vi "Data_Save_Initialisation.vi"() -> (2 "Initialisation":string[](array[string]))   [LabVIEW 2017]
uses:
  Ctrls/CSV_Data.ctl
panel:
  in  "Data in":T1
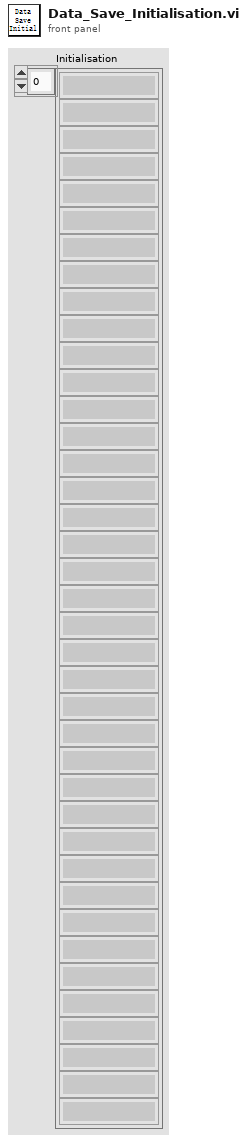
[diagram p1: front panel]
types:
  T1 = typedef "CSV_Data.ctl" = cluster{"Initialisation":cluster{"LMT - Connect UUT (con COM)":cluster{"Vaule":string, "Status":string, "Step Time":dbl}, "LMT - Software Version (rrel)":cluster{"Vaule":string, "Status":string, "Step Time":dbl}, "LMT - Write SKU file (wskuc)":cluster{"Vaule":string, "Status":string, "Step Time":dbl}, "LMT - SKU file name":cluster{"Vaule":string, "Status":string, "Step Time":dbl}, "LMT Connect UUT - Error Log":cluster{"Vaule":string, "Status":string, "Step Time":dbl}, "5.3.2.1 Connect UUT DDM":cluster{"Vaule":string, "Status":string, "Step Time":dbl}, "Connect UUT DDM - Error Log":cluster{"Vaule":string, "Status":string, "Step Time":dbl}, "5.3.2.8 Read DDM EOL Timestamp":cluster{"Vaule":string, "Status":string, "Step Time":dbl}, "5.3.2.8 Read DDM EOL Timestamp - Mode":cluster{"Vaule":string, "Status":string, "Step Time":dbl}, "5.3.2.8 Read DDM EOL Timestamp - Timestamp":cluster{"Vaule":string, "Status":string, "Step Time":dbl}, "5.3.2.8 Read DDM EOL Timestamp - Rig ID":cluster{"Vaule":string, "Status":string, "Step Time":dbl}, "5.3.2.8 Read DDM EOL Timestamp - Passmark ID":cluster{"Vaule":string, "Status":string, "Step Time":dbl}, "5.3.2.8 Read DDM EOL Timestamp - Passmark Rev":cluster{"Vaule":string, "Status":string, "Step Time":dbl}, "Read DDM EOL Timestamp - Error Log":cluster{"Vaule":string, "Status":string, "Step Time":dbl}, "5.3.2.2 Read DDM SW Version before flashing":cluster{"Vaule":string, "Status":string, "Step Time":dbl}, "5.3.2.2 Software Version before flashing":cluster{"Vaule":string, "Status":string, "Step Time":dbl}, "Read DDM SW Version before flashing - Error Log":cluster{"Vaule":string, "Status":string, "Step Time":dbl}, "5.3.2.7 Read Hardware Serial":cluster{"Vaule":string, "Status":string, "Step Time":dbl}, "Read Hardware Serial - Error Log":cluster{"Vaule":string, "Status":string, "Step Time":dbl}, "Read DDM SN from UUT":cluster{"Vaule":string, "Status":string, "Step Time":dbl}, "UUT DDM SN":cluster{"Vaule":string, "Status":string, "Step Time":dbl}, "Compare Length":cluster{"Vaule":string, "Status":string, "Step Time":dbl}, "Compare DDM SN with MES SN":cluster{"Vaule":string, "Status":string, "Step Time":dbl}, "Check DDM SN - Error Log":cluster{"Vaule":string, "Status":string, "Step Time":dbl}, "5.3.6.2.2 Backup File Data - CAL":cluster{"Vaule":string, "Status":string, "Step Time":dbl}, "5.3.6.2.2 Backup Data Response - CAL":cluster{"Vaule":string, "Status":string, "Step Time":dbl}, "5.3.2.3 Flash Firmware Version":cluster{"Vaule":string, "Status":string, "Step Time":dbl}, "5.3.2.4 Wait Timeout":cluster{"Vaule":string, "Status":string, "Step Time":dbl}, "5.3.2.5 Check SW Version":cluster{"Vaule":string, "Status":string, "Step Time":dbl}, "5.3.2.5 Flashing firmware file name":cluster{"Vaule":string, "Status":string, "Step Time":dbl}, "Flash Firmware Version - Error Log":cluster{"Vaule":string, "Status":string, "Step Time":dbl}, "5.3.2a.1 Disconnect UUT":cluster{"Vaule":string, "Status":string, "Step Time":dbl}, "Disconnect UUT - Error Log":cluster{"Vaule":string, "Status":string, "Step Time":dbl}, "5.3.2a.3 Connect UUT UI":cluster{"Vaule":string, "Status":string, "Step Time":dbl}, "Connect UUT UI - Error Log":cluster{"Vaule":string, "Status":string, "Step Time":dbl}, "5.3.2a.4 Flash Firmware Version":cluster{"Vaule":string, "Status":string, "Step Time":dbl}, "5.3.2a.4 Wait Timeout":cluster{"Vaule":string, "Status":string, "Step Time":dbl}, "5.3.2a.4 Check SW Version":cluster{"Vaule":string, "Status":string, "Step Time":dbl}, "5.3.2a.5 Flashing firmware file name":cluster{"Vaule":string, "Status":string, "Step Time":dbl}, "Flash Firmware Version - Error Log":cluster{"Vaule":string, "Status":string, "Step Time":dbl}, "5.3.2.6 Read DDM SW Version after flashing":cluster{"Vaule":string, "Status":string, "Step Time":dbl}, "5.3.2.6 Check DDM SW Version after flashing":cluster{"Vaule":string, "Status":string, "Step Time":dbl}, "Read DDM SW Version after flashing - Error Log":cluster{"Vaule":string, "Status":string, "Step Time":dbl}, "5.3.2.10 Set SKU Config Status":cluster{"Vaule":string, "Status":string, "Step Time":dbl}, "5.3.2.10 Set SKU Config":cluster{"Vaule":string, "Status":string, "Step Time":dbl}, "5.3.2.10 Set SKU Config File Name":cluster{"Vaule":string, "Status":string, "Step Time":dbl}, "Set SKU Config - Error Log":cluster{"Vaule":string, "Status":string, "Step Time":dbl}, "5.3.2.10 Ready Status":cluster{"Vaule":string, "Status":string, "Step Time":dbl}, "Ready Status - Error Log":cluster{"Vaule":string, "Status":string, "Step Time":dbl}, "5.3.2.12 Set Device Mode to EOL":cluster{"Vaule":string, "Status":string, "Step Time":dbl}, "5.3.2.12 DDM EOL mode":cluster{"Vaule":string, "Status":string, "Step Time":dbl}, "Set Device Mode - Error Log":cluster{"Vaule":string, "Status":string, "Step Time":dbl}, "5.3.4.34 Wait 1s":cluster{"Vaule":string, "Status":string, "Step Time":dbl}, "5.3.2.13 DDM Parameter - Voltage":cluster{"Vaule":string, "Status":string, "Step Time":dbl}, "5.3.2.13 DDM Parameter - Current":cluster{"Vaule":string, "Status":string, "Step Time":dbl}, "5.3.2.13 DDM Parameter - Power":cluster{"Vaule":string, "Status":string, "Step Time":dbl}, "5.3.2.13 DDM Parameter - Speed":cluster{"Vaule":string, "Status":string, "Step Time":dbl}, "5.3.2.13 DDM Parameter - Pressure":cluster{"Vaule":string, "Status":string, "Step Time":dbl}, "5.3.2.14 Tester Parameter - Voltage":cluster{"Vaule":string, "Status":string, "Step Time":dbl}, "5.3.2.14 Tester Parameter - Current":cluster{"Vaule":string, "Status":string, "Step Time":dbl}, "5.3.2.14 Tester Parameter - Power":cluster{"Vaule":string, "Status":string, "Step Time":dbl}, "5.3.2.14 Tester Parameter - Ambient Pressure":cluster{"Vaule":string, "Status":string, "Step Time":dbl}, "5.3.2.14 Tester Parameter - Ambient Temperature":cluster{"Vaule":string, "Status":string, "Step Time":dbl}, "5.3.2.14 Tester Parameter - Pressure Box":cluster{"Vaule":string, "Status":string, "Step Time":dbl}, "5.3.2.14 Tester Parameter - Reference Ambient Pressure":cluster{"Vaule":string, "Status":string, "Step Time":dbl}, "5.3.2.15 Calculated Parameter - DDM Pressure Corrected":cluster{"Vaule":string, "Status":string, "Step Time":dbl}, "5.3.2.15 Calculated Parameter - DDM Real Power":cluster{"Vaule":string, "Status":string, "Step Time":dbl}, "5.3.2.15 Calculated Parameter - Delta V":cluster{"Vaule":string, "Status":string, "Step Time":dbl}, "Get and Check Parameter - Error Log":cluster{"Vaule":string, "Status":string, "Step Time":dbl}}, "BEMF_Calibration":cluster{"5.3.3.0 Read BEMF ambient temperature":cluster{"Vaule":string, "Status":string, "Step Time":dbl}, "5.3.3.0 Calibration Result - eol_cold_bemf_temp":cluster{"Vaule":string, "Status":string, "Step Time":dbl}, "Read BEMF ambient temperature - Error Log":cluster{"Vaule":string, "Status":string, "Step Time":dbl}, "5.3.3.0 Set ambient temp to DDM":cluster{"Vaule":string, "Status":string, "Step Time":dbl}, "5.3.3.0 DDM Ambient Temp":cluster{"Vaule":string, "Status":string, "Step Time":dbl}, "Set ambient temp to DDM - Error Log":cluster{"Vaule":string, "Status":string, "Step Time":dbl}, "5.3.4.2 Restriction Plate Diameter":cluster{"Vaule":string, "Status":string, "Step Time":dbl}, "5.3.4.2 BEMF CAL - Put 13mm Restriction Plate":cluster{"Vaule":string, "Status":string, "Step Time":dbl}, "Put Restriction Plate - Error Log":cluster{"Vaule":string, "Status":string, "Step Time":dbl}, "5.3.3.1 Set - Calibrate BEMF both":cluster{"Vaule":string, "Status":string, "Step Time":dbl}, "5.3.3.1 Get - Calibrate BEMF LSI":cluster{"Vaule":string, "Status":string, "Step Time":dbl}, "5.3.3.2 Get - Calibration Result - eol_bemf_mp_cold_coef_a":cluster{"Vaule":string, "Status":string, "Step Time":dbl}, "5.3.3.2 Get - Calibration Result - eol_bemf_mp_cold_coef_b":cluster{"Vaule":string, "Status":string, "Step Time":dbl}, "5.3.3.2 Get - Calibration Result - eol_bemf_mp_cold_coef_c":cluster{"Vaule":string, "Status":string, "Step Time":dbl}, "5.3.3.2 Get - Calibration Result - eol_bemf_lsi_cold_ref_coeffs":cluster{"Vaule":string, "Status":string, "Step Time":dbl}, "5.3.3.2 Get - Calibration Result - eol_bemf_lsi_speed":cluster{"Vaule":string, "Status":string, "Step Time":dbl}, "5.3.3.2 Get - Calibration Result - eol_bemf_lsi_integral_0":cluster{"Vaule":string, "Status":string, "Step Time":dbl}, "5.3.3.2 Get - Calibration Result - eol_bemf_lsi_integral_1":cluster{"Vaule":string, "Status":string, "Step Time":dbl}, "5.3.3.2 Get - Calibration Result - eol_bemf_lsi_integral_2":cluster{"Vaule":string, "Status":string, "Step Time":dbl}, "5.3.3.2 Get - Calibration Result - eol_cold_bemf":cluster{"Vaule":string, "Status":string, "Step Time":dbl}, "5.3.3.2 Get - Calibration Result - eol_cold_bemf_fisf":cluster{"Vaule":string, "Status":string, "Step Time":dbl}, "Get - Calibrate BEMF LSI - Error Log":cluster{"Vaule":string, "Status":string, "Step Time":dbl}, "5.3.3.3 Finalise Calibration":cluster{"Vaule":string, "Status":string, "Step Time":dbl}, "5.3.3.4 Wait 1 sec":cluster{"Vaule":string, "Status":string, "Step Time":dbl}, "Finalise Calibration - Error Log":cluster{"Vaule":string, "Status":string, "Step Time":dbl}, "5.3.3.1 Get - Calibrate BEMF LSI":cluster{"Vaule":string, "Status":string, "Step Time":dbl}, "5.3.3.2 Get - Calibration Result - eol_cold_bemf":cluster{"Vaule":string, "Status":string, "Step Time":dbl}, "5.3.3.2 Get - Calibration Result - eol_cold_bemf_fisf":cluster{"Vaule":string, "Status":string, "Step Time":dbl}, "5.3.3.2 Compare -Calibration Result - eol_cold_bemf":cluster{"Vaule":string, "Status":string, "Step Time":dbl}, "5.3.3.2 Compare -Calibration Result - eol_cold_bemf_fisf":cluster{"Vaule":string, "Status":string, "Step Time":dbl}, "Get & Compare - Calibrate BEMF LSI - Error Log":cluster{"Vaule":string, "Status":string, "Step Time":dbl}}, "ECO":cluster{"5.3.3.3 Reset Power Tune":cluster{"Vaule":string, "Status":string, "Step Time":dbl}, "5.3.3.4 Reset Power Tune Value":cluster{"Vaule":string, "Status":string, "Step Time":dbl}, "Reset Power Tune - Error Log":cluster{"Vaule":string, "Status":string, "Step Time":dbl}, "5.3.3.3 Reset BEMF FISF Calibration":cluster{"Vaule":string, "Status":string, "Step Time":dbl}, "5.3.3.4 Reset BEMF FISF Calibration Value":cluster{"Vaule":string, "Status":string, "Step Time":dbl}, "Reset BEMF FISF Calibration - Error Log":cluster{"Vaule":string, "Status":string, "Step Time":dbl}, "5.3.4.2 ECO - Put 13mm Restriction Plate":cluster{"Vaule":string, "Status":string, "Step Time":dbl}, "5.3.4.2 Restriction Plate Diameter":cluster{"Vaule":string, "Status":string, "Step Time":dbl}, "Put Restriction Plate - Error Log":cluster{"Vaule":string, "Status":string, "Step Time":dbl}, "5.3.4.5 ECO - Motor ON":cluster{"Vaule":string, "Status":string, "Step Time":dbl}, "5.3.4.5 ECO - Motor ON Mode":cluster{"Vaule":string, "Status":string, "Step Time":dbl}, "ECO - Motor ON - Error Log":cluster{"Vaule":string, "Status":string, "Step Time":dbl}, "5.3.4.6 ECO - Motor Speed Stabilisation":cluster{"Vaule":string, "Status":string, "Step Time":dbl}, "5.3.4.6 ECO - Stabilisation Time":cluster{"Vaule":string, "Status":string, "Step Time":dbl}, "ECO - Motor Speed Stabilisation - Error Log":cluster{"Vaule":string, "Status":string, "Step Time":dbl}, "5.3.4.7 ECO - DDM Parameter - Voltage":cluster{"Vaule":string, "Status":string, "Step Time":dbl}, "5.3.4.7 ECO - DDM Parameter - Current":cluster{"Vaule":string, "Status":string, "Step Time":dbl}, "5.3.4.7 ECO - DDM Parameter - Power":cluster{"Vaule":string, "Status":string, "Step Time":dbl}, "5.3.4.7 ECO - DDM Parameter - Measured Power":cluster{"Vaule":string, "Status":string, "Step Time":dbl}, "5.3.4.7 ECO - DDM Parameter - Speed":cluster{"Vaule":string, "Status":string, "Step Time":dbl}, "5.3.4.7 ECO - DDM Parameter - Pressure":cluster{"Vaule":string, "Status":string, "Step Time":dbl}, "5.3.4.7 ECO - DDM Parameter - lsi magnet temp":cluster{"Vaule":string, "Status":string, "Step Time":dbl}, "5.3.4.7 ECO - DDM Parameter - fisf magnet temp":cluster{"Vaule":string, "Status":string, "Step Time":dbl}, "5.3.4.7 ECO - DDM Parameter - iir magnet temp":cluster{"Vaule":string, "Status":string, "Step Time":dbl}, "5.3.4.8 ECO - Tester Parameter - Voltage":cluster{"Vaule":string, "Status":string, "Step Time":dbl}, "5.3.4.8 ECO - Tester Parameter - Current":cluster{"Vaule":string, "Status":string, "Step Time":dbl}, "5.3.4.8 ECO - Tester Parameter - Power":cluster{"Vaule":string, "Status":string, "Step Time":dbl}, "5.3.4.8 ECO - Tester Parameter - Ambient Pressure":cluster{"Vaule":string, "Status":string, "Step Time":dbl}, "5.3.4.8 ECO - Tester Parameter - Ambient Temperature":cluster{"Vaule":string, "Status":string, "Step Time":dbl}, "5.3.4.8 ECO - Tester Parameter - Ambient Humidity":cluster{"Vaule":string, "Status":string, "Step Time":dbl}, "5.3.4.8 ECO - Tester Parameter - Pressure Box":cluster{"Vaule":string, "Status":string, "Step Time":dbl}, "5.3.4.8 ECO - Tester Parameter - Reference Ambient Pressure":cluster{"Vaule":string, "Status":string, "Step Time":dbl}, "5.3.4.9 ECO - Calculated Parameter - DDM Pressure Corrected":cluster{"Vaule":string, "Status":string, "Step Time":dbl}, "5.3.4.9 ECO - Calculated Parameter - DDM Real Power":cluster{"Vaule":string, "Status":string, "Step Time":dbl}, "5.3.4.9 ECO - Calculated Parameter - Delta V":cluster{"Vaule":string, "Status":string, "Step Time":dbl}, "5.3.4.9 ECO - Calculated Parameter - Flowrate":cluster{"Vaule":string, "Status":string, "Step Time":dbl}, "5.3.4.9 ECO - Calculated Parameter - Airwatt":cluster{"Vaule":string, "Status":string, "Step Time":dbl}, "5.3.4.9 ECO - Formula":cluster{"Vaule":string, "Status":string, "Step Time":dbl}, "ECO - Get and Check Parameter - Error Log":cluster{"Vaule":string, "Status":string, "Step Time":dbl}, "PT ECO - Power Tune Mode Status":cluster{"Vaule":string, "Status":string, "Step Time":dbl}, "PT ECO - Power Tune Set Delta Power Tune":cluster{"Vaule":string, "Status":string, "Step Time":dbl}, "PT ECO - Power Tune Index":cluster{"Vaule":string, "Status":string, "Step Time":dbl}, "PT ECO - Power Tune Delta_P":cluster{"Vaule":string, "Status":string, "Step Time":dbl}, "PT ECO - Power Tune Motor ON Status":cluster{"Vaule":string, "Status":string, "Step Time":dbl}, "PT ECO - Power Tune Motor ON Mode":cluster{"Vaule":string, "Status":string, "Step Time":dbl}, "PT ECO - Power Tune Stabilisation Time Status":cluster{"Vaule":string, "Status":string, "Step Time":dbl}, "PT ECO - Power Tune Stabilisation Delay Time":cluster{"Vaule":string, "Status":string, "Step Time":dbl}, "PT ECO - DDM Parameter - Voltage":cluster{"Vaule":string, "Status":string, "Step Time":dbl}, "PT ECO - DDM Parameter - Current":cluster{"Vaule":string, "Status":string, "Step Time":dbl}, "PT ECO - DDM Parameter - Power":cluster{"Vaule":string, "Status":string, "Step Time":dbl}, "PT ECO - DDM Parameter - Measured Power":cluster{"Vaule":string, "Status":string, "Step Time":dbl}, "PT ECO - DDM Parameter - Speed":cluster{"Vaule":string, "Status":string, "Step Time":dbl}, "PT ECO - DDM Parameter - Pressure":cluster{"Vaule":string, "Status":string, "Step Time":dbl}, "PT ECO - DDM Parameter - lsi magnet temp":cluster{"Vaule":string, "Status":string, "Step Time":dbl}, "PT ECO - DDM Parameter - fisf magnet temp":cluster{"Vaule":string, "Status":string, "Step Time":dbl}, "PT ECO - DDM Parameter - iir magnet temp":cluster{"Vaule":string, "Status":string, "Step Time":dbl}, "PT ECO - Tester Parameter - Voltage":cluster{"Vaule":string, "Status":string, "Step Time":dbl}, "PT ECO - Tester Parameter - Current":cluster{"Vaule":string, "Status":string, "Step Time":dbl}, "PT ECO - Tester Parameter - Power":cluster{"Vaule":string, "Status":string, "Step Time":dbl}, "PT ECO - Tester Parameter - Ambient Pressure":cluster{"Vaule":string, "Status":string, "Step Time":dbl}, "PT ECO - Tester Parameter - Ambient Temperature":cluster{"Vaule":string, "Status":string, "Step Time":dbl}, "PT ECO - Tester Parameter - Ambient Humidity":cluster{"Vaule":string, "Status":string, "Step Time":dbl}, "PT ECO - Tester Parameter - Pressure Box":cluster{"Vaule":string, "Status":string, "Step Time":dbl}, "PT ECO - Tester Parameter - Reference Ambient Pressure":cluster{"Vaule":string, "Status":string, "Step Time":dbl}, "PT ECO - Calculated Parameter - DDM Pressure Corrected":cluster{"Vaule":string, "Status":string, "Step Time":dbl}, "PT ECO - Calculated Parameter - DDM Real Power":cluster{"Vaule":string, "Status":string, "Step Time":dbl}, "PT ECO - Calculated Parameter - Delta V":cluster{"Vaule":string, "Status":string, "Step Time":dbl}, "PT ECO - Calculated Parameter - Flowrate":cluster{"Vaule":string, "Status":string, "Step Time":dbl}, "PT ECO - Calculated Parameter - Airwatt":cluster{"Vaule":string, "Status":string, "Step Time":dbl}, "PT ECO - Formula":cluster{"Vaule":string, "Status":string, "Step Time":dbl}, "PT ECO - Get and Check Parameter - Error Log":cluster{"Vaule":string, "Status":string, "Step Time":dbl}}, ...}
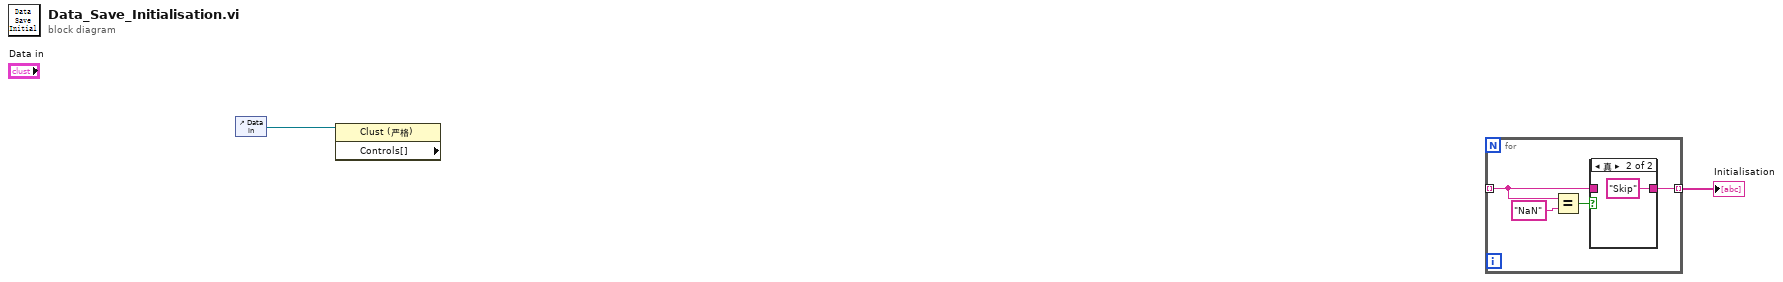
[diagram p0: block diagram]
diagram:
  n1 = control-ref of="Data in"() -> (w1:refnum<vi>)
  n2 = property class="Clust (严格)" props=["Controls[]"](reference=w1) -> ()  [unwired: 1 in, 3 out]
  n3 = for {
    tunnel: [w7] -> w2 mode=indexing
    tunnel: [w4] -> w3 mode=indexing
    n4 = Equal?(x=w4, y="NaN" ("x")) -> (x = y?=w5:bool)
    n5 = case shown="真" w5 {
      tunnel: [w8 "Skip" ("x")] -> w7
      tunnel: w4 -> [w8 _]
      frame False {
      }
      frame True {
      }
    }
  }
  "Initialisation" <- w2
